vi "auto_placeblock.vi"(11 "Chain IN":bool) -> (3 "Chain OUT":bool)   [LabVIEW 2010, in "LASA Beta.lvrbt"]
uses:
  LASA Beta.lvrbt
  op-run.vi
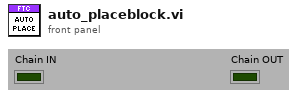
[diagram p1: front panel]
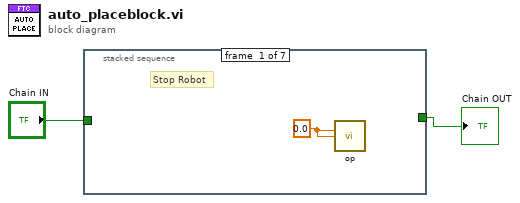
[diagram p0: block diagram]
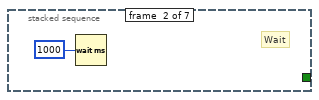
[diagram p2: hidden frame]
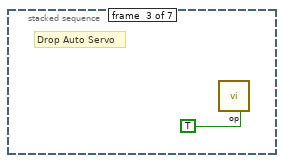
[diagram p3: hidden frame]
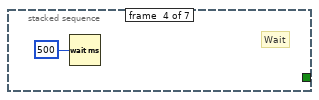
[diagram p4: hidden frame]
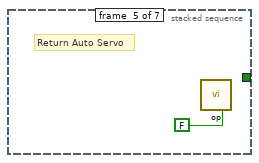
[diagram p5: hidden frame]
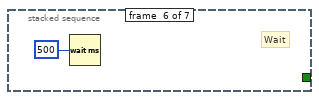
[diagram p6: hidden frame]
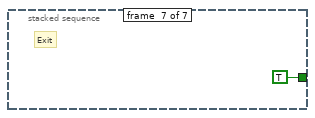
[diagram p7: hidden frame]
diagram:
  n1 = stacked-sequence {
    tunnel: [_ _ _ _ _ _ TRUE] -> w2
    tunnel: "Chain IN" -> [_ _ _ _ _ _ _]
    frame #0 {
      w3 = 0.0 ("Left Drive")
      # "Stop Robot"
      n2 = call-poly "op.vi"("Left Drive"=w3, "Right Drive"=w3) -> ()  [unwired: 13 in, 1 out]
    }
    frame #1 {
      # "Wait"
      n3 = Wait (ms)(milliseconds to wait=u32 1000) -> ()  [unwired: 1 out]
    }
    frame #2 {
      # "Drop Auto Servo"
      n4 = call-poly "op.vi"("Auto Servo"=TRUE) -> ()  [unwired: 14 in, 1 out]
    }
    frame #3 {
      # "Wait"
      n5 = Wait (ms)(milliseconds to wait=u32 500) -> ()  [unwired: 1 out]
    }
    frame #4 {
      # "Return Auto Servo"
      n6 = call-poly "op.vi"("Auto Servo"=FALSE) -> ()  [unwired: 14 in, 1 out]
    }
    frame #5 {
      # "Wait"
      n7 = Wait (ms)(milliseconds to wait=u32 500) -> ()  [unwired: 1 out]
    }
    frame #6 {
      # "Exit"
    }
  }
  "Chain OUT" <- w2
